vi "Pockels-manage mod setting.vi"(8 "error in (no error)":errorcluster, 10 "Function":enum16{"Capture setting", "Re-apply setting"}(ring)) -> (0 "error out":errorcluster)   [LabVIEW 2017]
uses:
  Globals/gl_Pockels control globals.vi
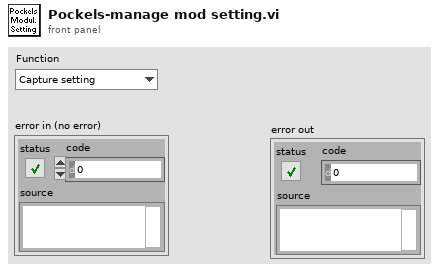
[diagram p1: front panel]
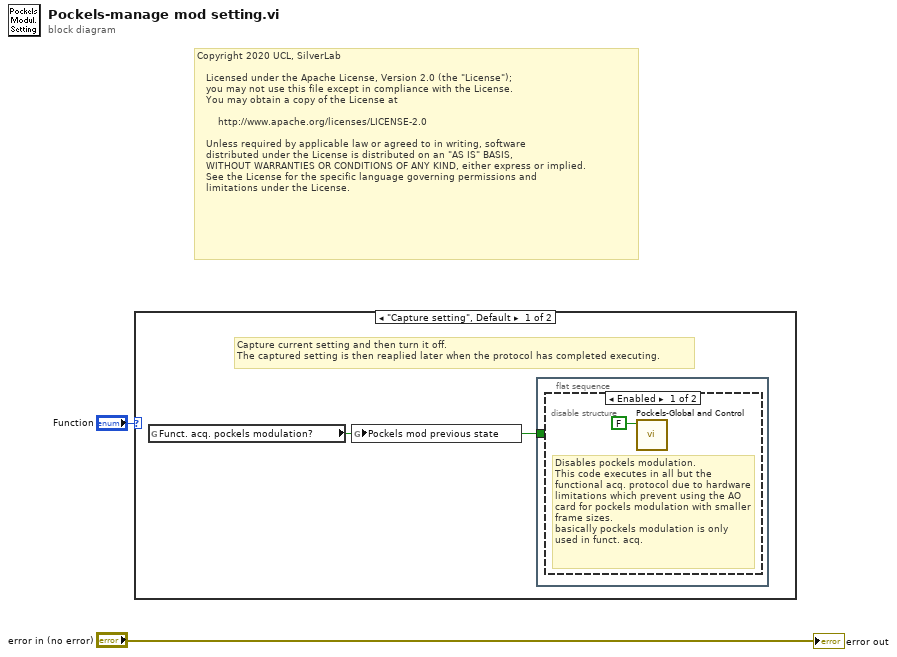
[diagram p0: block diagram]
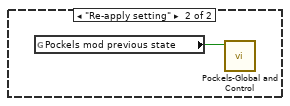
[diagram p3: hidden frame]
diagram:
  # "Copyright 2020 UCL, SilverLab\n \n   Licensed under the Apache License, Version 2.0 (the \"License\");\n   you may not use this file except in compliance with the License.\n   You may obtain a copy of the License at\n \n       http://www.apache.org/licenses/LICENSE-2.0\n \n   Unless required by applicable law or agreed to in writing, software\n   distributed under the License is distributed on an \"AS IS\" BASIS,\n   WITHOUT WARRANTIES OR CONDITIONS OF ANY KIND, either express or implied.\n   See the License for the specific language governing permissions and\n   limitations under the License."
  n1 = case shown="\"Capture setting\", Default" "Function" {
    frame "Capture setting", Default {
      # "Capture current setting and then turn it off.\nThe captured setting is then reaplied later when the protocol has completed executing."
      n2 = global read "gl_Pockels control globals.vi" "Funct. acq. pockels modulation?"() -> (w3:bool)
      n3 = global write "gl_Pockels control globals.vi" "Pockels mod previous state"(w3) -> ()
      n4 = flat-sequence {
        tunnel: w3 -> [_]
        frame #0 {
          n5 = disable-structure shown="Enabled" {
            frame Enabled {
              # "Disables pockels modulation.\nThis code executes in all but the functional acq. protocol due to hardware limitations which prevent using the AO card for pockels modulation with smaller frame sizes.\nbasically pockels modulation is only used in funct. acq."
              n6 = call "Pockels-Global and Control.vi"("Pockels modulation is ON"=FALSE) -> ()  [unwired: 11 in]
            }
            frame Disabled {
            }
          }
        }
      }
    }
    frame "Re-apply setting" {
      n7 = global read "gl_Pockels control globals.vi" "Pockels mod previous state"() -> (w5:bool)
      n8 = call "Pockels-Global and Control.vi"("Pockels modulation is ON"=w5) -> ()  [unwired: 11 in]
    }
  }
  "error out" <- "error in (no error)"
